vi "CRYUpdate Unicode Caption.vi"(5 "Interpret as Unicode (T)":bool=TRUE, 6 "error in (no error)":errorcluster, 7 "Caption":string="\u0000\u0000\u0000\u0000", 9 "Control Reference":refnum<vi>) -> (0 "error out":errorcluster, 3 "Control Reference":refnum<vi>)   [LabVIEW 2013]
doc: "Apply a caption text to the specified control/indicator. Interpret string as Unicode is set."
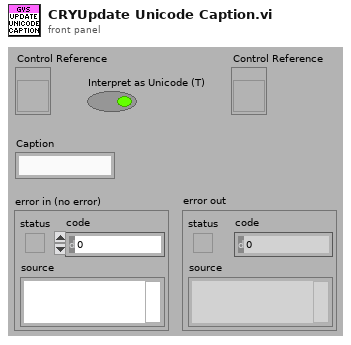
[diagram p1: front panel]
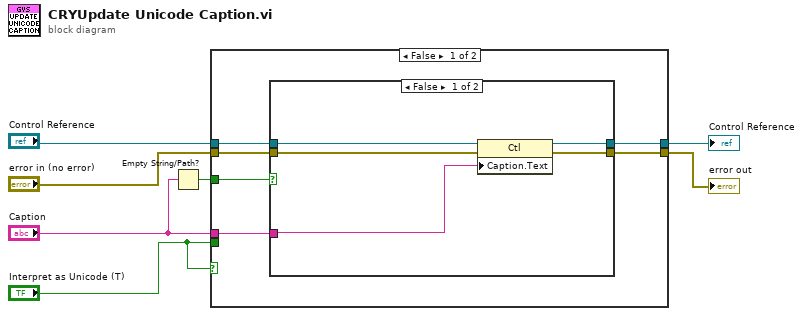
[diagram p0: block diagram]
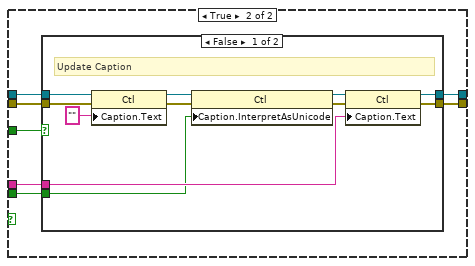
[diagram p3: hidden frame]
diagram:
  n1 = Empty String/Path?(string/path="Caption") -> (empty?=w6:bool)
  n2 = case shown="False" "Interpret as Unicode (T)" {
    tunnel: "error in (no error)" -> [w9 w27]
    tunnel: w6 -> [w13 w26]
    tunnel: "Caption" -> [w12 w25]
    tunnel: "Interpret as Unicode (T)" -> [_ w24]
    tunnel: "Control Reference" -> [w10 w23]
    tunnel: [w8 w22] -> w3
    tunnel: [w11 w21] -> w2
    frame False {
      n3 = case shown="False" w13 {
        tunnel: w12 -> [w18 _]
        tunnel: [w17 w20] -> w11
        tunnel: w10 -> [w16 w20]
        tunnel: w9 -> [w15 w19]
        tunnel: [w14 w19] -> w8
        frame False {
          n4 = property class="Ctl"(reference=w16, error in=w15, "Caption.Text"=w18) -> (reference out=w17:refnum<vi>, error out=w14:errorcluster)
        }
        frame True {
        }
      }
    }
    frame True {
      n5 = case shown="False" w26 {
        tunnel: w23 -> [w36 w40]
        tunnel: w27 -> [w33 w39]
        tunnel: w25 -> [w32 _]
        tunnel: [w38 w40] -> w21
        tunnel: [w37 w39] -> w22
        tunnel: w24 -> [w30 _]
        frame False {
          # "Update Caption"
          n6 = property class="Ctl"(reference=w36, error in=w33, "Caption.Text"="") -> (reference out=w35:refnum<vi>, error out=w34:errorcluster)
          n7 = property class="Ctl"(reference=w35, error in=w34, "Caption.InterpretAsUnicode"=w30) -> (reference out=w29:refnum<vi>, error out=w28:errorcluster)
          n8 = property class="Ctl"(reference=w29, error in=w28, "Caption.Text"=w32) -> (reference out=w38:refnum<vi>, error out=w37:errorcluster)
        }
        frame True {
        }
      }
    }
  }
  "error out" <- w3
  "Control Reference" <- w2
